vi "FRCts20_Backend_INI_Write_Revision.vi"(8 "error in (no error)":errorcluster, 9 "Save? (T)":bool=TRUE, 10 "Revision":T1={"Major Revision"=1, "Minor Revision"=1, "Branch Number"=1, "Build Phase"="a", "Build Number"=1}, 11 "INI Controller in":refnum<class "FRCts20_Backend_INI Controller.lvclass">) -> (0 "error out":errorcluster, 3 "INI Controller out":refnum<class "FRCts20_Backend_INI Controller.lvclass">)   [LabVIEW 2014, in "FRCts20_Backend_Engine.lvlib" / "FRCts20_Backend_INI Controller.lvclass"]
uses:
  FRCts20_Backend_INI Controller.lvclass
  FRCts20_Backend_INI_Revision.ctl
  FRCts20_Backend_INI Controller.lvclass/FRCts20_Backend_INI Controller.ctl
  <vilib>/Utility/config.llb/Write Key (String).vi
  <vilib>/Utility/config.llb/NI_LVConfig.lvlib
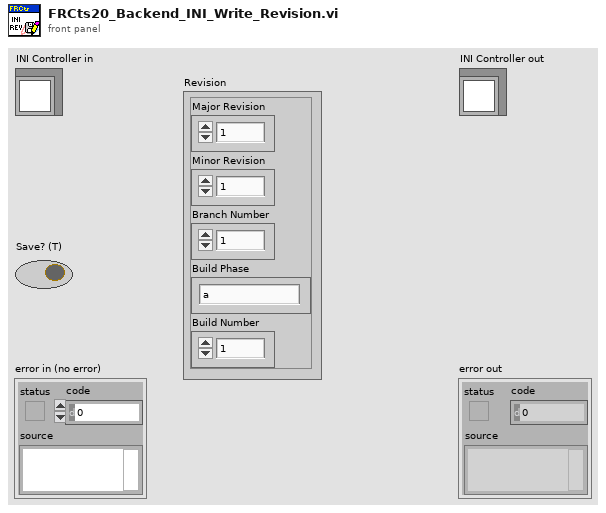
[diagram p1: front panel]
types:
  T1 = typedef "FRCts20_Backend_Engine.lvlib/FRCts20_Backend_INI Controller.lvclass/FRCts20_Backend_INI_Revision.ctl" = cluster{"Major Revision":i32, "Minor Revision":i32, "Branch Number":i32, "Build Phase":string, "Build Number":i32}
  T2 = typedef "NI_LVConfig.lvlib/Config Data RefNum.ctl" = refnum<k1>
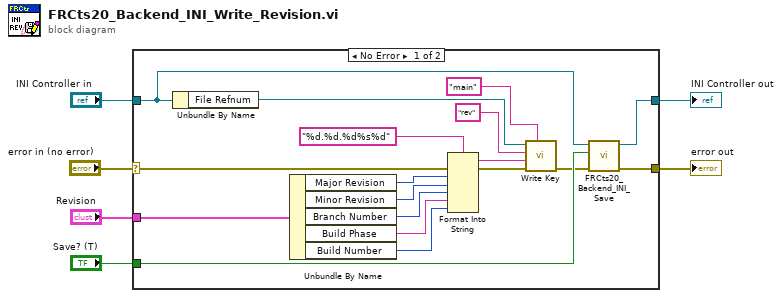
[diagram p0: block diagram]
diagram:
  n1 = case shown="No Error" "error in (no error)" {
    selector: "error in (no error)" -> [w8 w25]
    tunnel: [w23 w25] -> w5
    tunnel: [w22 w26] -> w3
    tunnel: "INI Controller in" -> [w21 w26]
    tunnel: "Save? (T)" -> [w24 _]
    tunnel: "Revision" -> [w14 _]
    frame No Error {
      n2 = Unbundle By Name(w21) -> ("File Refnum"=w18:T2)
      n3 = Unbundle By Name(w14) -> ("Major Revision"=w9:i32, "Minor Revision"=w10:i32, "Branch Number"=w11:i32, "Build Phase"=w13:string, "Build Number"=w12:i32)
      n4 = Format Into String(format string="%d.%d.%d%s%d", error in=w8, w9, w10, w11, w13, w12) -> (resulting string=w7:string, error out=w16:errorcluster)  [unwired: 1 in]
      n5 = call-poly <vilib>:"Write Key.vi"("section"="main", "error in (no error)"=w16, "value"=w7, "key"="rev", "refnum"=w18) -> ("error out"=w17:errorcluster)  [unwired: 4 in, 2 out]
      n6 = call "FRCts20_Backend_INI_Save.vi"("error in (no error)"=w17, "Save? (T)"=w24, "INI Controller in"=w21) -> ("error out"=w23:errorcluster, "INI Controller out"=w22:refnum<class "FRCts20_Backend_INI Controller.lvclass">)  [unwired: 7 in]
    }
    frame Error {
    }
  }
  "error out" <- w5
  "INI Controller out" <- w3
